vi "System.vi"(8 "error in (no error)":errorcluster, 11 "Node Ptr":T4 format="%.0x") -> (0 "error out":errorcluster)   [LabVIEW 2016, in "DCM System Explorer.lvlib"]
uses:
  DCM System Explorer.lvlib
  <vilib>/NI Veristand/Custom Device API/Custom Device Item Ref.ctl
  <vilib>/Powertrain Controls/Device Drivers/DCM/Rev0/RT/System Settings.ctl
  <vilib>/Powertrain Controls/Device Drivers/DCM/Rev0/RT/User LED.ctl
  <vilib>/Powertrain Controls/Device Drivers/DCM/HH/RT/Duration Pre Scale.ctl
  Shared/DCM Properties.vi
  Shared/DCM Constants and GUIDs.vi
  <vilib>/NI Veristand/Custom Device Tools/Custom Device Utility Library/NI VeriStand - Search for Item by Name.vi
  <vilib>/NI VeriStand/Custom Device API/Custom Device API.lvlib
  DCM Shared.lvlib
  <vilib>/NI Veristand/Custom Device Tools/Custom Device Utility Library/Custom Device Utility Library.lvlib
  <vilib>/Powertrain Controls/Device Drivers/DCM/Rev0/RT/DCM - RT.lvclass
  <vilib>/Powertrain Controls/Device Drivers/DCM/HH/RT/DCM - RT - HH.lvlib
panel:
  in  "System Settings":T1 {"HH Open Threshold [A]" min=0 max=8 format="%#_3p"; "HH ISeq Dur PS" items=["3.3ms @ 20MHz"=0, "6.5ms @ 10MHz"=4, "13ms @ 5MHz"=6, "26ms @ 2.5MHz"=7]; "HH Shoot Through Time [s]" min=0 max=0.003277 format="%#_3p"; "Clamp Fault Filter Time [s]" min=0 max=0.003277 format="%#_3p"; "DI HS Fault Filter Time [s]" min=0 max=0.003277 format="%#_3p"}
  in  "Header":cluster{"Section Name":string}={"Section Name"="System Initial Settings"}
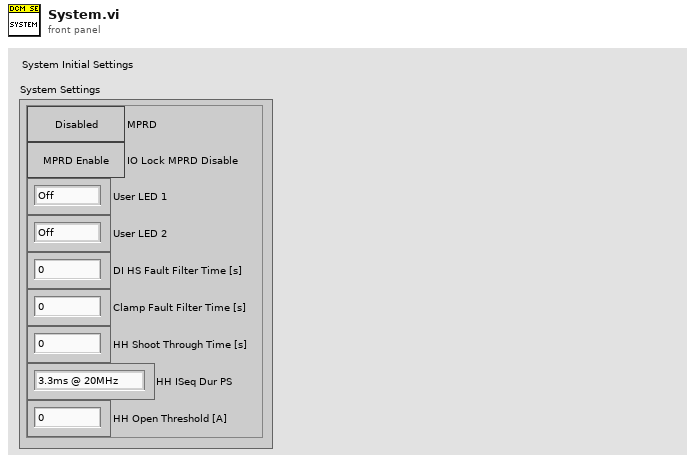
[diagram p1: front panel]
types:
  T1 = typedef "DCM - RT.lvclass/System Settings.ctl" = cluster{"MPRD":bool, "IO Lock MPRD Disable":bool, "User LED 1":T2, "User LED 2":T2, "DI HS Fault Filter Time [s]":sgl, "Clamp Fault Filter Time [s]":sgl, "HH Shoot Through Time [s]":sgl, "HH ISeq Dur PS":T3, "HH Open Threshold [A]":sgl}
  T2 = typedef "DCM - RT.lvclass/User LED.ctl" = enum16{"Off", "Yellow", "Green"}
  T3 = typedef "DCM - RT - HH.lvlib/Duration Pre Scale.ctl" = u8
  T4 = typedef "Custom Device API.lvlib/Custom Device Item Ref.ctl" = u64
  T5 = typedef "Custom Device API.lvlib/Custom Device Commands.ctl" = enum16{"Default", "Item renamed", "Shutdown", "Dynamic button pressed"}
  T6 = typedef "DCM Shared.lvlib/Channel.ctl" = cluster{"Name":string, "Units":string, "Default":dbl, "Description":string}
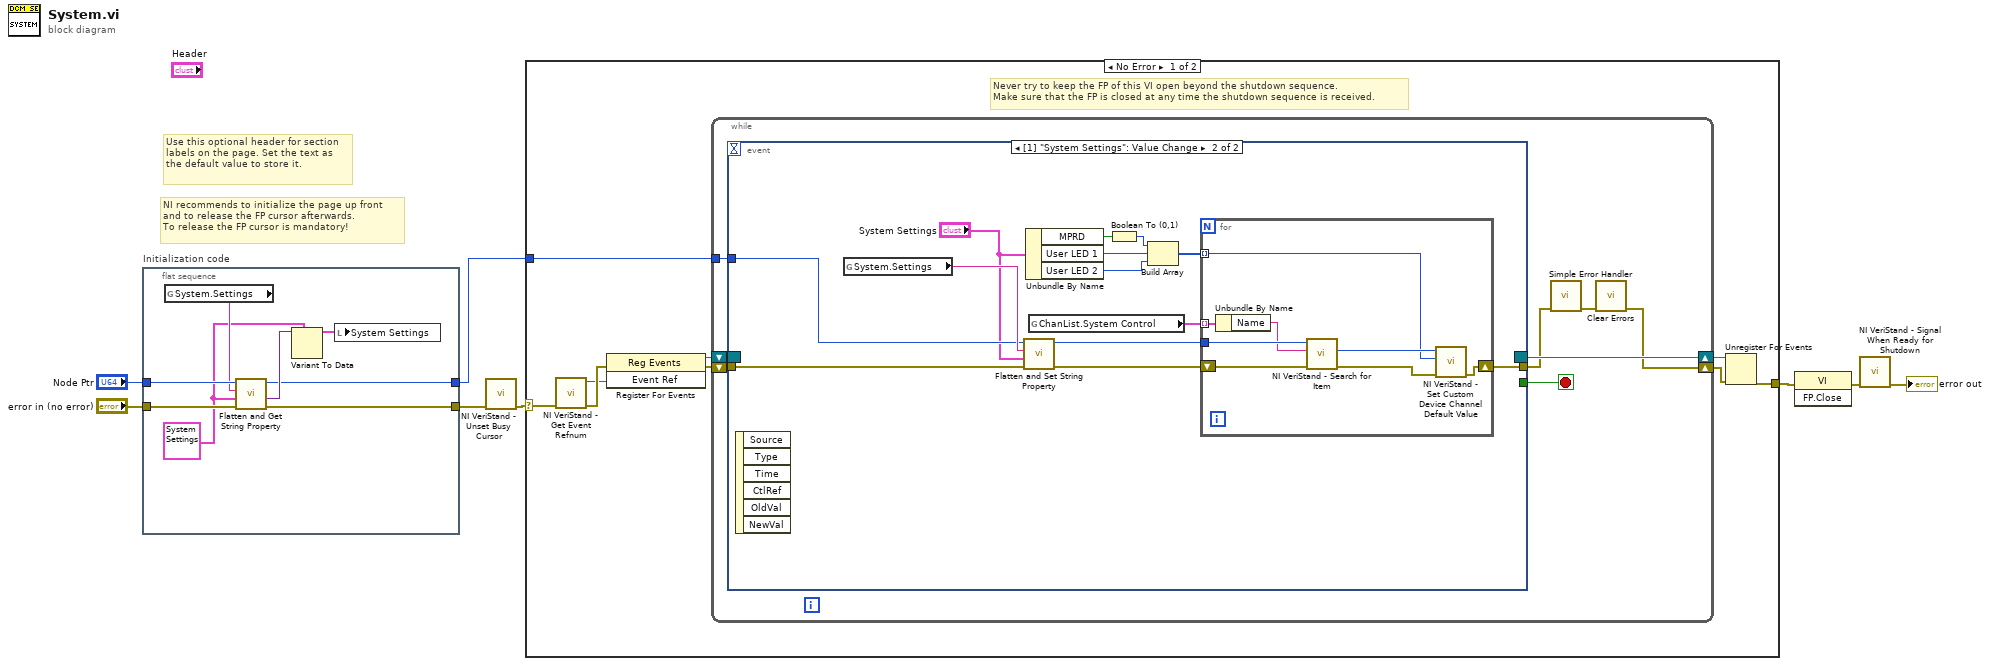
[diagram p0: block diagram]
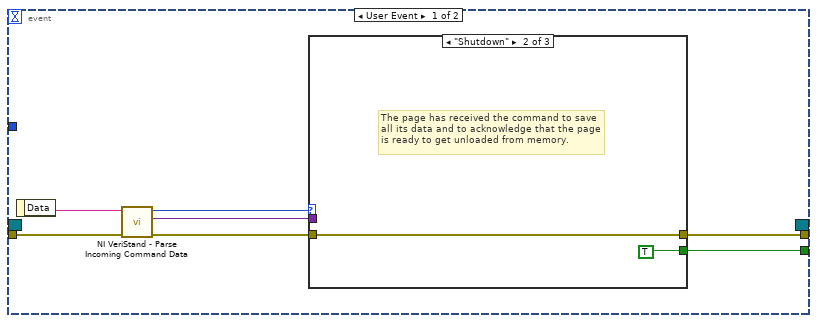
[diagram p2: hidden frame]
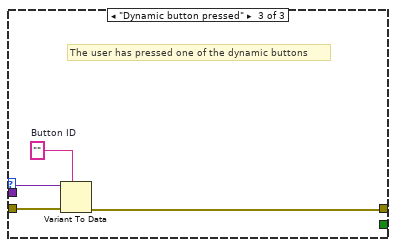
[diagram p4: hidden frame]
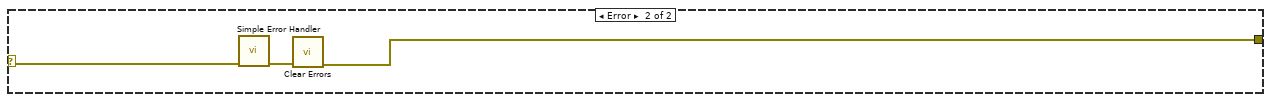
[diagram p5: hidden frame]
diagram:
  # "Use this optional header for section labels on the page. Set the text as the default value to store it."
  # "NI recommends to initialize the page up front\nand to release the FP cursor afterwards.\nTo release the FP cursor is mandatory!"
  n1 = flat-sequence "Initialization code" {
    tunnel: "error in (no error)" -> [w16]
    tunnel: "Node Ptr" -> [w15]
    tunnel: [w11] -> w2
    tunnel: [w12] -> w1
    frame #0 {
      w10 = T1 {"MPRD"=FALSE, "IO Lock MPRD Disable"=FALSE, "User LED 1"=enum."Off", "User LED 2"=enum."Off", "DI HS Fault Filter Time [s]"=0.0, "Clamp Fault Filter Time [s]"=0.0, "HH Shoot Through Time [s]"=0.0, "HH ISeq Dur PS"=0, "HH Open Threshold [A]"=0.0} ("System Settings")
      n2 = global read "DCM Properties.vi" "System.Settings"() -> (w13:string)
      n3 = call "Flatten and Get String Property.vi"("error in (no error)"=w16, "Default Value"=w10, "Property Name"=w13, "Section Ref in"=w15) -> ("error out"=w12:errorcluster, "Value"=w14:variant, "Section Ref out"=w11:T4)  [unwired: 5 in]
      n4 = Variant To Data(type=w10, Variant=w14) -> (data=w9:T1)  [unwired: 1 in, 1 out]
      n5 = local write "System Settings"(w9) -> ()
    }
  }
  n6 = call <vilib>:"NI VeriStand - Unset Busy Cursor.vi"("error in (no error)"=w1) -> ("error out"=w4:errorcluster)  [unwired: 10 out]
  n7 = case shown="No Error" w4 {
    selector: w4 -> [w18 w71]
    tunnel: [w22 w69] -> w8
    tunnel: w2 -> [w17 _]
    frame No Error {
      # "Never try to keep the FP of this VI open beyond the shutdown sequence.\nMake sure that the FP is closed at any time the shutdown sequence is received."
      n8 = call <vilib>:"NI VeriStand - Get Event Refnum.vi"("error in (no error)"=w18) -> ("error out"=w25:errorcluster, "Event Ref"=w21:refnum<user-event>)  [unwired: 9 out]
      n9 = register-events(error in=w25, w21) -> (reference out=w19:refnum<event-registration>, error out=w20:errorcluster)  [unwired: 1 in]
      n10 = while {
        shift-right: [w27] -> w23
        shift-left: w20 -> [w32]
        shift-right: [w33] -> w24
        shift-left: w19 -> [w31]
        tunnel: w17 -> [w26]
        stop <- w30 stop-if-true
        n11 = event shown="[1] \"System Settings\": Value Change" {
          selector: w31 -> [_ _]
          dyn-events: [_ _] -> w33
          timeout: _ -> [_ _]
          tunnel: w32 -> [w40 w48]
          tunnel: [w36 _] -> w30
          tunnel: [w35 w51] -> w29
          tunnel: w26 -> [_ w50]
          event User Event {
            n12 = event-data() -> ("Data"=w39:string)  [unwired: 1 out]
            n13 = call <vilib>:"NI VeriStand - Parse Incoming Command Data.vi"("error in (no error)"=w40, "Incoming data"=w39) -> ("error out"=w38:errorcluster, "Outgoing data"=w34:variant, "Action"=w37:T5)  [unwired: 7 out]
            n14 = case shown="\"Shutdown\"" w37 {
              tunnel: w38 -> [w41 w42 w47]
              tunnel: [_ TRUE _] -> w36
              tunnel: [w41 w42 w44] -> w35
              tunnel: w34 -> [_ _ w46]
              frame "Default", Default {
              }
              frame "Shutdown" {
                # "The page has received the command to save all its data and to acknowledge that the page is ready to get unloaded from memory."
              }
              frame "Dynamic button pressed" {
                w45 = ""  # Button ID
                # "The user has pressed one of the dynamic buttons"
                n15 = Variant To Data(error in=w47, type=w45, Variant=w46) -> (error out=w44:errorcluster)  [unwired: 1 out]
              }
            }
          }
          event Value Change {
            n16 = event-data() -> ()  [unwired: 7 out]
            n17 = global read "DCM Properties.vi" "System.Settings"() -> (w60:string)
            n18 = call "Flatten and Set String Property.vi"("error in (no error)"=w48, "Value"="System Settings", "Property Name"=w60, "Section Ref in"=w50) -> ("error out"=w58:errorcluster, "Section Ref out"=w59:T4)  [unwired: 6 in]
            n19 = Unbundle By Name("System Settings") -> ("MPRD"=w56:bool, "User LED 1"=w54:T2, "User LED 2"=w53:T2)
            n20 = global read "DCM Constants and GUIDs.vi" "ChanList.System Control"() -> (w57:T6[])
            n21 = Boolean To (0,1)(Boolean=w56) -> (0, 1=w55:i16)
            n22 = Build Array(w55, w54, w53) -> (w52:u16[])
            n23 = for {
              tunnel: w59 -> [w68]
              tunnel: w57 -> [w66] mode=indexing
              shift-right: [w62] -> w51
              shift-left: w58 -> [w67]
              tunnel: w52 -> [w61] mode=indexing
              n24 = Unbundle By Name(w66) -> ("Name"=w65:string)
              n25 = call-poly <vilib>:"NI VeriStand - Search for Item.vi"("error in"=w67, "Item Name"=w65, "Section Ref in"=w68) -> ("error out"=w63:errorcluster, "Item Ref"=w64:T4)  [unwired: 5 in, 2 out]
              n26 = call <vilib>:"NI VeriStand - Set Custom Device Channel Default Value.vi"("error in (no error)"=w63, "Default Value"=w61, "Channel Ref in"=w64) -> ("error out"=w62:errorcluster)  [unwired: 7 in, 1 out]
            }
          }
        }
        n27 = call <vilib>:"Simple Error Handler.vi"("error in (no error)"=w29) -> ("error out"=w28:errorcluster)  [unwired: 1 in, 7 out]
        n28 = call <vilib>:"Clear Errors.vi"("error in (no error)"=w28) -> ("error out"=w27:errorcluster)  [unwired: 1 in, 5 out]
      }
      n29 = Unregister For Events(event registration refnum=w24, error in=w23) -> (error out=w22:errorcluster)
    }
    frame Error {
      n30 = call <vilib>:"Simple Error Handler.vi"("error in (no error)"=w71) -> ("error out"=w70:errorcluster)  [unwired: 1 in, 7 out]
      n31 = call <vilib>:"Clear Errors.vi"("error in (no error)"=w70) -> ("error out"=w69:errorcluster)  [unwired: 1 in, 5 out]
    }
  }
  n32 = invoke class="VI" method="FP.Close"(error in=w8) -> (error out=w7:errorcluster)  [unwired: 2 in, 2 out]
  n33 = call <vilib>:"NI VeriStand - Signal When Ready for Shutdown.vi"("error in (no error)"=w7) -> ("error out"=→"error out":errorcluster)  [unwired: 10 out]
